vi "Pre Launch Init.vi"(11 "PCC in":refnum<class "PCC.lvclass">) -> (0 "error out":errorcluster, 3 "PCC out":refnum<class "PCC.lvclass">)   [LabVIEW 2018, in "PCC Actor.lvlib" / "PCC.lvclass"]
doc: "(<B>Filename</B>: Actor Framework.lvlib:Actor.lvclass:Pre Launch Init.vi)\n\nDefines behavior that occurs after the Launch Nested Actor method is invoked but before the actor's Actor Core method begins running.\n\nBy default, this method does nothing. A descendant class may override it to define behavior."
uses:
  PCC.lvclass
  C:/Users/Administrator/Desktop/2018LabVIEW EMS/IED Actors/Device DDS Communications Framework/Device DDS Communications/Device DDS Communications.lvclass
  C:/Users/Administrator/Desktop/2018LabVIEW EMS/EMS Generic Actor/EMS Generic/EMS Generic.lvclass
  Device DDS Communications Framework/Device DDS Communications/Device DDS Communications.lvclass/Device DDS Communications.ctl
  <vilib>/ORNL/CSEISMIC DDS/CSEISMIC DDS Base/CSEISMIC DDS.lvclass/CSEISMIC DDS.ctl
  <vilib>/ORNL/CSEISMIC DDS/CSEISMIC DDS Base/Accessors/Write DDS Reference.vi
  <vilib>/ORNL/CSEISMIC DDS/DDS Writer/DDS Writer.lvclass
  C:/Program Files (x86)/National Instruments/LabVIEW 2018/vi.lib/ORNL/CSEISMIC DDS/CSEISMIC DDS Base/CSEISMIC DDS.lvclass
  <vilib>/ORNL/CSEISMIC DDS/CSEISMIC DDS Base/Error Handler.vi
  Device DDS Communications Framework/Device DDS Communications/Device DDS Communications.lvclass
  EMS Generic Actor/EMS Generic/EMS Generic.lvclass
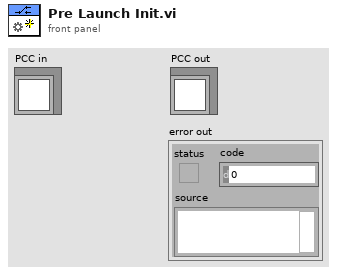
[diagram p1: front panel]
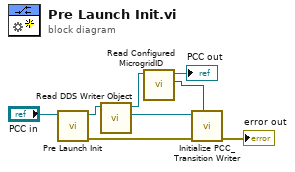
[diagram p0: block diagram]
diagram:
  n1 = call-parent "Pre Launch Init.vi"("Device DDS Communications in"="PCC in") -> ("error out"=w1:errorcluster, "Device DDS Communications out"=w3:refnum<class "PCC.lvclass">)  [unwired: 9 in]
  n2 = call "Read DDS Writer Object.vi"("Device DDS Communications in"=w3) -> ("DDS Writer Object"=w7:refnum<class "DDS Writer.lvclass">, "Device DDS Communications out"=w8:refnum<class "PCC.lvclass">)  [unwired: 9 in]
  n3 = call "Read Configured MicrogridID.vi"("EMS Generic in"=w8) -> ("Microgrid ID"=w6:u8, "EMS Generic out"=→"PCC out":refnum<class "PCC.lvclass">)  [unwired: 8 in, 1 out]
  n4 = call <vilib>:"Initialize PCC_Transition Writer.vi"("MicrogridID"=w6, "error in"=w1, "DDS Writer in"=w7) -> ("error out"=→"error out":errorcluster)  [unwired: 7 in, 1 out]
